vi "compute sum.vi"(8 "error in (no error)":errorcluster, 9 "Roy":u8[][](array[numeric]), 10 "Rob":u8[][](array[numeric]), 11 "Thorcam in":refnum<class "Thorcam.lvclass">) -> (0 "error out":errorcluster, 3 "Thorcam out":refnum<class "Thorcam.lvclass">)   [LabVIEW 2012, in "Thorcam.lvclass"]
uses:
  Thorcam.lvclass
  Thorcam.lvclass/Thorcam.ctl
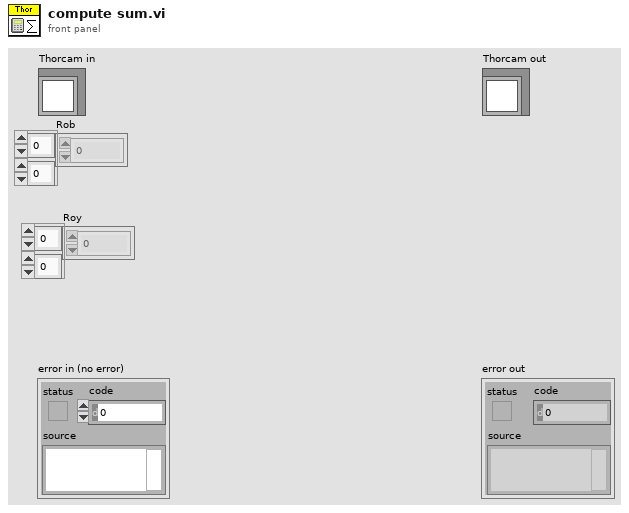
[diagram p1: front panel]
types:
  T1 = cluster{"x dimension":i32, "mean":dbl, "standard deviation":dbl, "y dimension":i32}
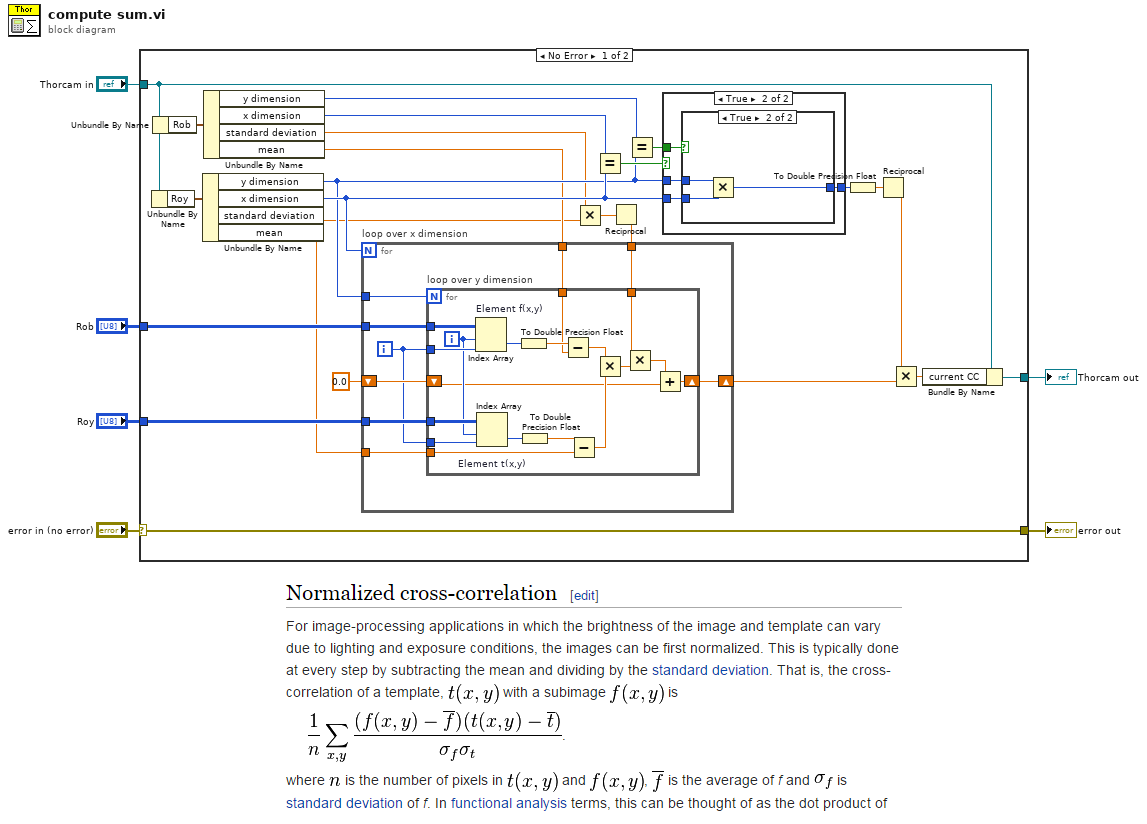
[diagram p0: block diagram]
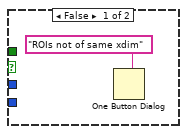
[diagram p2: hidden frame]
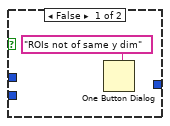
[diagram p3: hidden frame]
diagram:
  n1 = case shown="No Error" "error in (no error)" {
    selector: "error in (no error)" -> [w31 w69]
    tunnel: [w31 w69] -> w5
    tunnel: [w7 w68] -> w3
    tunnel: "Thorcam in" -> [w8 w68]
    tunnel: "Rob" -> [w25 _]
    tunnel: "Roy" -> [w18 _]
    frame No Error {
      n2 = Unbundle By Name(w8) -> ("Roy"=w29:T1)
      n3 = Unbundle By Name(w8) -> ("Rob"=w30:T1)
      n4 = Unbundle By Name(w29) -> ("y dimension"=w19:i32, "x dimension"=w20:i32, "standard deviation"=w13:dbl, "mean"=w12:dbl)
      n5 = Unbundle By Name(w30) -> ("y dimension"=w22:i32, "x dimension"=w28:i32, "standard deviation"=w15:dbl, "mean"=w14:dbl)
      n6 = Multiply(x=w15, y=w13) -> (x*y=w17:dbl)
      n7 = Equal?(x=w28, y=w20) -> (x = y?=w23:bool)
      n8 = Reciprocal(x=w17) -> (1/x=w16:dbl)
      n9 = for "loop over x dimension" {
        N: w20 -> [_]
        tunnel: w19 -> [w40]
        tunnel: w25 -> [w39]
        tunnel: w14 -> [w38]
        shift-right: [w37] -> w10
        shift-left: 0.0 -> [w36]
        tunnel: w18 -> [w35]
        tunnel: w12 -> [w33]
        tunnel: w16 -> [w32]
        i -> [w34]
        n10 = for "loop over y dimension" {
          N: w40 -> [_]
          tunnel: w39 -> [w58]
          tunnel: w34 -> [w57]
          tunnel: w38 -> [w54]
          shift-right: [w53] -> w37
          shift-left: w36 -> [w41]
          tunnel: w35 -> [w51]
          tunnel: w34 -> [w50]
          tunnel: w33 -> [w47]
          tunnel: w32 -> [w43]
          i -> [w49]
          n11 = Index Array "Element f(x,y)"(array=w58, index (row)=w49, index (col)=w57) -> (element=w56:u8)
          n12 = Index Array "Element t(x,y)"(array=w51, index (row)=w49, index (col)=w50) -> (element=w52:u8)
          n13 = To Double Precision Float(number=w56) -> (double precision float=w55:dbl)
          n14 = To Double Precision Float(number=w52) -> (double precision float=w48:dbl)
          n15 = Subtract(x=w55, y=w54) -> (x-y=w45:dbl)
          n16 = Subtract(x=w48, y=w47) -> (x-y=w46:dbl)
          n17 = Multiply(x=w45, y=w46) -> (x*y=w44:dbl)
          n18 = Multiply(x=w43, y=w44) -> (x*y=w42:dbl)
          n19 = Add(x=w42, y=w41) -> (x+y=w53:dbl)
        }
      }
      n20 = Equal?(x=w22, y=w19) -> (x = y?=w21:bool)
      n21 = case shown="True" w23 {
        tunnel: w20 -> [_ w61]
        tunnel: [_ w60] -> w26
        tunnel: w21 -> [_ w63]
        tunnel: w19 -> [_ w62]
        frame False {
          n22 = One Button Dialog(message="ROIs not of same xdim") -> ()  [unwired: 1 in, 1 out]
        }
        frame True {
          n23 = case shown="True" w63 {
            tunnel: w62 -> [_ w67]
            tunnel: w61 -> [_ w66]
            tunnel: [_ w65] -> w60
            frame False {
              n24 = One Button Dialog(message="ROIs not of same y dim") -> ()  [unwired: 1 in, 1 out]
            }
            frame True {
              n25 = Multiply(x=w67, y=w66) -> (x*y=w65:i32)
            }
          }
        }
      }
      n26 = To Double Precision Float(number=w26) -> (double precision float=w27:dbl)
      n27 = Reciprocal(x=w27) -> (1/x=w11:dbl)
      n28 = Multiply(x=w11, y=w10) -> (x*y=w9:dbl)
      n29 = Bundle By Name(cluster=w8, "current CC"=w9) -> (w7:refnum<class "Thorcam.lvclass">)
    }
    frame Error {
    }
  }
  "error out" <- w5
  "Thorcam out" <- w3
